vi "AIT 1553 - Create DB Bus Parm Config from Sysdef Tree.vi"(0 "Device Ptr":u64, 9 "Bus":T1, 11 "error in":errorcluster) -> (4 "Device Ptr dup":u64, 10 "Bus Out":T1, 15 "error out":errorcluster)   [LabVIEW 2013]
uses:
  Controls/1553_Bus.ctl
  Controls/1553_Bus_Controller.ctl
  Controls/1553_BC_Message.ctl
  Controls/1553 Param.ctl
  Controls/1553_Acyclic_Frame.ctl
  Controls/1553_Bus_Monitor.ctl
  Controls/1553_BM_Message.ctl
  Controls/1553_RT_Message.ctl
  <vilib>/NI Veristand/Custom Device API/Custom Device Item Ref.ctl
  <vilib>/NI Veristand/Custom Device Tools/Custom Device Utility Library/Search Direction.ctl
  Controls and Global/Global.vi
  <vilib>/NI Veristand/Custom Device Tools/Custom Device Utility Library/NI VeriStand - Search for Item by GUID.vi
  AIT 1553 Custom Device.lvlib
  <vilib>/NI Veristand/Custom Device Tools/Custom Device Utility Library/Custom Device Utility Library.lvlib
  <vilib>/NI Veristand/Custom Device API/Custom Device API.lvlib
panel:
  out "Item Ref":T9 format="%.0x"
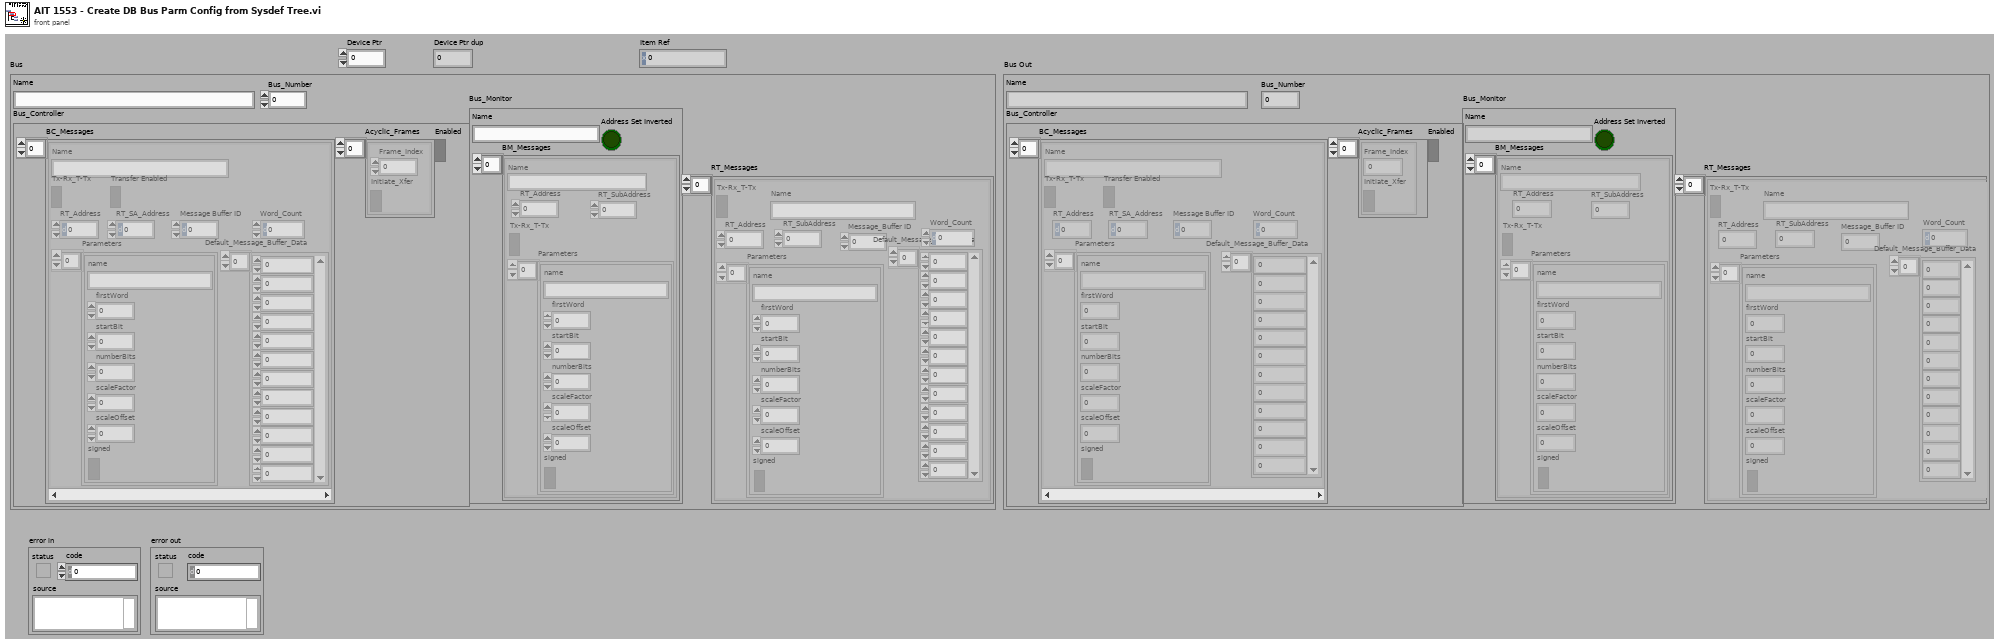
[diagram p1: front panel]
types:
  T1 = typedef "AIT 1553 Custom Device.lvlib/1553_Bus.ctl" = cluster{"Name":string, "Bus_Number":u8, "Bus_Controller":T2, "Bus_Monitor":T6, "RT_Messages":T8[]}
  T2 = typedef "AIT 1553 Custom Device.lvlib/1553_Bus_Controller.ctl" = cluster{"BC_Messages":T3[], "Acyclic_Frames":T5[], "Enabled":bool}
  T3 = typedef "AIT 1553 Custom Device.lvlib/1553_BC_Message.ctl" = cluster{"Name":string, "Tx-Rx_T-Tx":bool, "RT_Address":u8, "RT_SA_Address":u8, "Parameters":T4[], "Transfer Enabled":bool, "Message Buffer ID":u16, "Default_Message_Buffer_Data":u16[], "Word_Count":u8}
  T4 = typedef "AIT 1553 Custom Device.lvlib/1553 Param.ctl" = cluster{"name":string, "firstWord":i32, "startBit":i32, "numberBits":i32, "scaleFactor":dbl, "scaleOffset":dbl, "signed":bool}
  T5 = typedef "AIT 1553 Custom Device.lvlib/1553_Acyclic_Frame.ctl" = cluster{"Frame_Index":u8, "Initiate_Xfer":bool}
  T6 = typedef "AIT 1553 Custom Device.lvlib/1553_Bus_Monitor.ctl" = cluster{"Name":string, "BM_Messages":T7[], "Address Set Inverted":bool}
  T7 = typedef "AIT 1553 Custom Device.lvlib/1553_BM_Message.ctl" = cluster{"RT_Address":u8, "RT_SubAddress":u8, "Tx-Rx_T-Tx":bool, "Parameters":T4[], "Name":string}
  T8 = typedef "AIT 1553 Custom Device.lvlib/1553_RT_Message.ctl" = cluster{"RT_Address":u8, "RT_SubAddress":u8, "Tx-Rx_T-Tx":bool, "Parameters":T4[], "Message_Buffer ID":u16, "Default_Message_Buffer_Data":u16[], "Word_Count":u8, "Name":string}
  T9 = typedef "Custom Device API.lvlib/Custom Device Item Ref.ctl" = u64
  T10 = typedef "Custom Device Utility Library.lvlib/Search Direction.ctl" = enum16{"Down", "Up"}
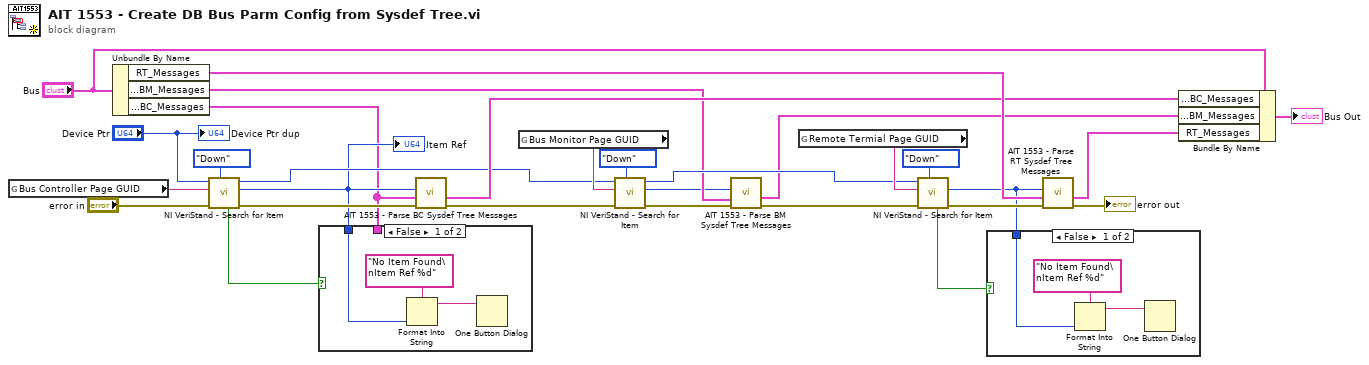
[diagram p0: block diagram]
diagram:
  n1 = global read "Global.vi" "Bus Controller Page GUID"() -> (w28:string)
  n2 = Unbundle By Name("Bus") -> ("RT_Messages"=w21:T8[], "Bus_Monitor.BM_Messages"=w7:T7[], "Bus_Controller.BC_Messages"=w1:T3[])
  n3 = call-poly <vilib>:"NI VeriStand - Search for Item.vi"("Direction (Down)"=Search_Direction."Down", "error in"="error in", "Item GUID"=w28, "Section Ref in"="Device Ptr") -> ("error out"=w27:errorcluster, "Item Ref"=w2:T9, "Section Ref out"=w4:T9, "Found"=w25:bool)  [unwired: 4 in]
  "Item Ref" <- w2
  n4 = case shown="False" w25 {
    tunnel: w2 -> [w31 _]
    tunnel: w1 -> [_ _]
    frame False {
      n5 = Format Into String(format string="No Item Found\nItem Ref %d" ("message"), w31) -> (resulting string=w30:string)  [unwired: 2 in, 1 out]
      n6 = One Button Dialog(message=w30) -> ()  [unwired: 1 in, 1 out]
    }
    frame True {
    }
  }
  n7 = call "AIT 1553 - Parse BC Sysdef Tree Messages.vi"("error in"=w27, "BC Messages In"=w1, "Section Ptr"=w2) -> ("error out"=w12:errorcluster, "BC Messages Out"=w14:T3[])  [unwired: 7 in]
  n8 = global read "Global.vi" "Bus Monitor Page GUID"() -> (w11:string)
  n9 = call-poly <vilib>:"NI VeriStand - Search for Item.vi"("Direction (Down)"=Search_Direction."Down", "error in"=w12, "Item GUID"=w11, "Section Ref in"=w4) -> ("error out"=w9:errorcluster, "Item Ref"=w6:T9, "Section Ref out"=w10:T9)  [unwired: 4 in, 1 out]
  n10 = call "AIT 1553 - Parse BM Sysdef Tree Messages.vi"("error in"=w9, "BM_Messages In"=w7, "Section Ptr"=w6) -> ("error out"=w8:errorcluster, "BM_Messages Out"=w3:T7[])  [unwired: 7 in]
  n11 = global read "Global.vi" "Remote Termial Page GUID"() -> (w23:string)
  n12 = call-poly <vilib>:"NI VeriStand - Search for Item.vi"("Direction (Down)"=Search_Direction."Down", "error in"=w8, "Item GUID"=w23, "Section Ref in"=w10) -> ("error out"=w22:errorcluster, "Item Ref"=w17:T9, "Found"=w18:bool)  [unwired: 4 in, 1 out]
  n13 = case shown="False" w18 {
    tunnel: w17 -> [w34 _]
    frame False {
      n14 = Format Into String(format string="No Item Found\nItem Ref %d" ("message"), w34) -> (resulting string=w33:string)  [unwired: 2 in, 1 out]
      n15 = One Button Dialog(message=w33) -> ()  [unwired: 1 in, 1 out]
    }
    frame True {
    }
  }
  n16 = call "AIT 1553 - Parse RT Sysdef Tree Messages.vi"("error in"=w22, "RT_Messages"=w21, "Section Ptr"=w17) -> ("error out"=→"error out":errorcluster, "RT_Messages Out"=w5:T8[])  [unwired: 7 in]
  n17 = Bundle By Name(cluster="Bus", "Bus_Controller.BC_Messages"=w14, "Bus_Monitor.BM_Messages"=w3, "RT_Messages"=w5) -> (→"Bus Out":T1)
  "Device Ptr dup" <- "Device Ptr"
